vi "Get Mobile Platform.vi"(8 "error in (no error)":errorcluster, 11 "KUKA youBot host in":refnum<class "NI_Robotics_KUKA youBot Host Interface.lvclass">) -> (0 "error out":errorcluster, 2 "KUKA youBot platform out":refnum<class "NI_Robotics_KUKA youBot Platform.lvclass">, 3 "KUKA youBot host out":refnum<class "NI_Robotics_KUKA youBot Host Interface.lvclass">)   [LabVIEW 2017, in "NI_Robotics_KUKA youBot Host.lvlib" / "NI_Robotics_KUKA youBot Host Interface.lvclass"]
doc: "Returns a reference to the KUKA youBot mobile platform."
uses:
  <vilib>/robotics/KUKA youBot/Host Interface/NI_Robotics_KUKA youBot Host Interface.lvclass
  <vilib>/robotics/KUKA youBot/Basic Device/Mobile Platform/NI_Robotics_KUKA youBot Platform.lvclass
  <vilib>/robotics/KUKA youBot/Host Interface/NI_Robotics_KUKA youBot Host Interface.lvclass/NI_Robotics_KUKA youBot Host Interface.ctl
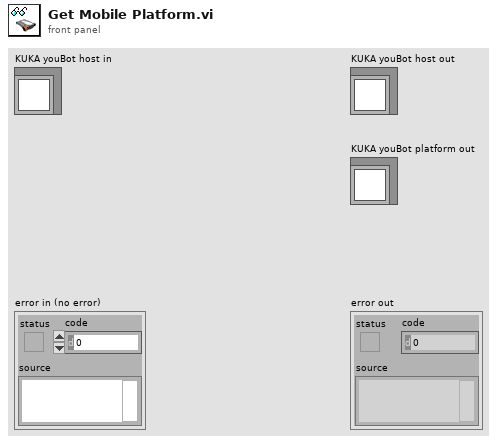
[diagram p1: front panel]
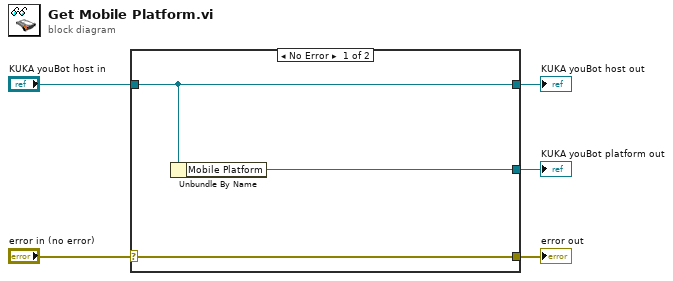
[diagram p0: block diagram]
diagram:
  n1 = case shown="No Error" "error in (no error)" {
    selector: "error in (no error)" -> [w8 w9]
    tunnel: [w8 w9] -> w4
    tunnel: [w7 w10] -> w2
    tunnel: "KUKA youBot host in" -> [w7 w10]
    tunnel: [w6 _] -> w1
    frame No Error {
      n2 = Unbundle By Name(w7) -> ("Mobile Platform"=w6:refnum<class "NI_Robotics_KUKA youBot Platform.lvclass">)
    }
    frame Error {
    }
  }
  "error out" <- w4
  "KUKA youBot host out" <- w2
  "KUKA youBot platform out" <- w1
